vi "-8211 Invalid Instrument Identifier--error.vi"(8 "error in":errorcluster, 11 "Source":string) -> (0 "error out":errorcluster)   [LabVIEW 2024, in "Instrument Manager.lvclass"]
uses:
  Instrument Manager.lvclass
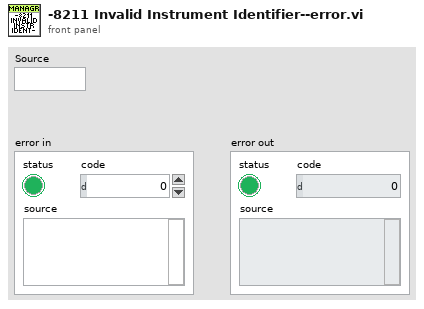
[diagram p1: front panel]
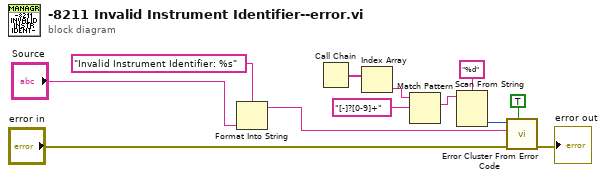
[diagram p0: block diagram]
diagram:
  n1 = Format Into String(format string="Invalid Instrument Identifier: %s", "Source") -> (resulting string=w11:string)  [unwired: 2 in, 1 out]
  n2 = Call Chain() -> (call chain=w6:string[])
  n3 = Index Array(array=w6) -> (element=w4:string)  [unwired: 1 in]
  n4 = Match Pattern(string=w4, regular expression="[-]?[0-9]+") -> (match substring=w3:string)  [unwired: 1 in, 3 out]
  n5 = Scan From String(format string="%d", input string=w3) -> (output 1=w1:i32)  [unwired: 3 in, 3 out]
  n6 = call <vilib>:"Error Cluster From Error Code.vi"("show call chain? (False)"=TRUE, "error in (no error)"="error in", "error message (\"\")"=w11, "error code (0)"=w1) -> ("error out"=→"error out":errorcluster)  [unwired: 5 in]
